vi "dfd_Generate Quantized Gain Report.vi"(8 "error in (no error)":errorcluster, 11 "filter in":T1={"mSRate_Fs"=1.0, "mSRate_Version"="1.0", "mSRate_Comments"="", "mSRate_OrgCoef"={"type"=enum."Undefined", "gain"=1.0, "coef a (k)"=[], "coef b (v)"=[]}, "mSRate_CurCoef"={"type"=enum."Undefined", "gain"=1.0, "coef a (k)"=[], "coef b (v)"=[]}, "mSRate_Quantized?"=FALSE, "mSRate_QCoef"={"type"=enum."Undefined", "gain"=1.0, "coef a (k)"=[], "coef b (v)"=[]}, "mSRate_QSettings"=[], "mSRate_Order"=0, "mSRate_Scaling"={"mSRate_ScaleByPowerOf2?"=FALSE, "mSRate_ScaleType"=enum."No Norm"}} {"mSRate_QSettings"."source" items=["Coef a/k"=0, "Coef b/v"=7, "Input"=1, "Output"=2, "Multiplicand"=3, "Product"=4, "Sum"=5, "Delay"=6, "Gain"=8]}) -> (0 "error out":errorcluster, 2 "gain report":string, 3 "filter out":T1={"mSRate_Fs"=1.0, "mSRate_Version"="1.0", "mSRate_Comments"="", "mSRate_OrgCoef"={"type"=enum."Undefined", "gain"=1.0, "coef a (k)"=[], "coef b (v)"=[]}, "mSRate_CurCoef"={"type"=enum."Undefined", "gain"=1.0, "coef a (k)"=[], "coef b (v)"=[]}, "mSRate_Quantized?"=FALSE, "mSRate_QCoef"={"type"=enum."Undefined", "gain"=1.0, "coef a (k)"=[], "coef b (v)"=[]}, "mSRate_QSettings"=[], "mSRate_Order"=0, "mSRate_Scaling"={"mSRate_ScaleByPowerOf2?"=FALSE, "mSRate_ScaleType"=enum."No Norm"}} {"mSRate_QSettings"."source" items=["Coef a/k"=0, "Coef b/v"=7, "Input"=1, "Output"=2, "Multiplicand"=3, "Product"=4, "Sum"=5, "Delay"=6, "Gain"=8]})   [LabVIEW 2017, in "NI_DigFilter_FXP.lvlib"]
uses:
  <vilib>/addons/Digital Filter Design/NI_DigFilter_FXP.lvlib
  <vilib>/addons/Digital Filter Design/_Objects.llb/DFD Filter Obj.ctl
  <vilib>/addons/Digital Filter Design/_Objects.llb/DFD Filter Coef.ctl
  <vilib>/addons/Digital Filter Design/_Objects.llb/DFD Filter Structure Type Selector.ctl
  <vilib>/addons/Digital Filter Design/_Objects.llb/dfd_Internal Quantization Settings.ctl
  <vilib>/addons/Digital Filter Design/_Objects.llb/dfd_Internal Quantization Srcs.ctl
  <vilib>/addons/Digital Filter Design/_Objects.llb/DFD Coef Norm Type.ctl
  <vilib>/addons/Digital Filter Design/NI_DigFilterLicensed.lvlib
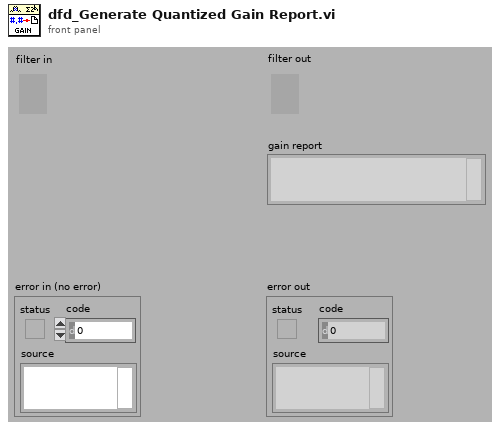
[diagram p1: front panel]
types:
  T1 = typedef "NI_DigFilterLicensed.lvlib/DFD Filter Obj.ctl" = cluster{"mSRate_Fs":dbl, "mSRate_Version":string, "mSRate_Comments":string, "mSRate_OrgCoef":T2, "mSRate_CurCoef":T2, "mSRate_Quantized?":bool, "mSRate_QCoef":T2, "mSRate_QSettings":T4[], "mSRate_Order":i32, "mSRate_Scaling":cluster{"mSRate_ScaleByPowerOf2?":bool, "mSRate_ScaleType":T6}}
  T2 = typedef "NI_DigFilterLicensed.lvlib/DFD Filter Coef.ctl" = cluster{"type":T3, "gain":dbl, "coef a (k)":dbl[], "coef b (v)":dbl[]}
  T3 = typedef "NI_DigFilterLicensed.lvlib/DFD Filter Structure Type Selector.ctl" = enum16{"Undefined", "FIR Direct Form", "FIR Direct Form Transposed", "FIR Symmetric", "FIR Antisymmetric", "IIR Direct Form I", "IIR Direct Form I Transposed", "IIR Direct Form II", "IIR Direct Form II Transposed", "IIR Cascaded Second Order Sections Form I", "IIR Cascaded Second Order Sections Form I Transposed", "IIR Cascaded Second Order Sections Form II", "IIR Cascaded Second Order Sections Form II Transposed", "Lattice Allpass (basic sections)", "Lattice Allpass (one multiplier sections)", "Lattice Allpass (normalized sections)", "Lattice AR (basic sections)", "Lattice AR (one multiplier sections)", "Lattice AR (normalized sections)", "Lattice MA (minimum phase)", "Lattice MA (maximum phase)", "Lattice ARMA (basic sections)", "Lattice ARMA (one multiplier sections)", "Lattice ARMA (normalized sections)"}
  T4 = typedef "NI_DigFilterLicensed.lvlib/dfd_Internal Quantization Settings.ctl" = cluster{"source":T5, "wl":i16, "iwl":i16, "overflow mode":enum16{"Saturation", "Wrap"}, "rounding mode":enum16{"Nearest", "Truncation"}, "signed?":bool}
  T5 = typedef "NI_DigFilterLicensed.lvlib/dfd_Internal Quantization Srcs.ctl" = u16
  T6 = typedef "NI_DigFilterLicensed.lvlib/DFD Coef Norm Type.ctl" = enum16{"No Norm", "Time Domain 1-Norm", "Time Domain 2-Norm", "Time Domain Inf-Norm"}
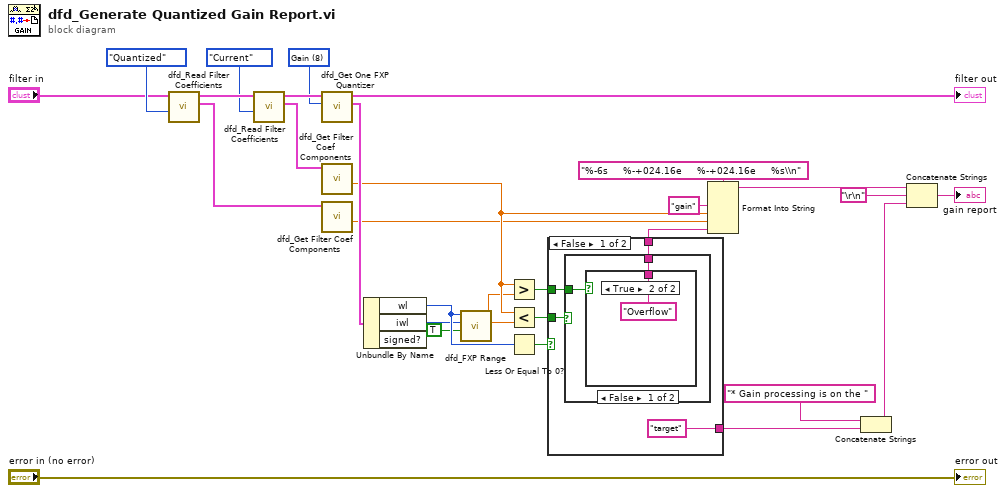
[diagram p0: block diagram]
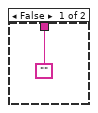
[diagram p2: hidden frame]
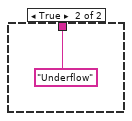
[diagram p3: hidden frame]
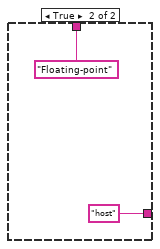
[diagram p4: hidden frame]
diagram:
  w19 = T5 8 items=["Coef a/k"=0, "Coef b/v"=7, "Input"=1, "Output"=2, "Multiplicand"=3, "Product"=4, "Sum"=5, "Delay"=6, "Gain"=8] ("quantization source")
  n1 = call <vilib>:"dfd_Read Filter Coefficients.vi"("coef source"=enum16{"Original", "Current", "Quantized"}."Quantized", "filter in"="filter in") -> ("filter coef"=w24:T2, "filter out"=w30:T1)  [unwired: 1 in, 7 out]
  n2 = call <vilib>:"dfd_Read Filter Coefficients.vi"("coef source"=enum16{"Original", "Current", "Quantized"}."Current", "filter in"=w30) -> ("filter coef"=w26:T2, "filter out"=w29:T1)  [unwired: 1 in, 7 out]
  n3 = call <vilib>:"dfd_Get One FXP Quantizer.vi"("quantization source"=w19, "filter in"=w29) -> ("quantization settings"=w23:T4, "filter out"=→"filter out":T1)  [unwired: 1 in, 7 out]
  n4 = call <vilib>:"dfd_Get Filter Coef Components.vi"("filter coef"=w26) -> ("gain"=w22:dbl)  [unwired: 1 in, 9 out]
  n5 = call <vilib>:"dfd_Get Filter Coef Components.vi"("filter coef"=w24) -> ("gain"=w21:dbl)  [unwired: 1 in, 9 out]
  n6 = Unbundle By Name(w23) -> ("wl"=w4:i16, "iwl"=w3:i16)  [unwired: 1 out]
  n7 = call <vilib>:"dfd_FXP Range.vi"("signed?"=TRUE, "iwl"=w3, "wl"=w4) -> ("low"=w18:ext, "high"=w17:ext)  [unwired: 7 out]
  n8 = Greater?(x=w22, y=w17) -> (0:w11:bool)
  n9 = Less?(x=w22, y=w18) -> (x < y?=w14:bool)
  n10 = Less Or Equal To 0?(x=w4) -> (x <= 0?=w12:bool)
  n11 = case shown="False" w12 {
    tunnel: w14 -> [w34 _]
    tunnel: [w33 "Floating-point"] -> w13
    tunnel: w11 -> [w32 _]
    tunnel: ["target" "host"] -> w9
    frame False {
      n12 = case shown="False" w34 {
        tunnel: [w36 "Underflow"] -> w33
        tunnel: w32 -> [w35 _]
        frame False {
          n13 = case shown="True" w35 {
            tunnel: ["" "Overflow"] -> w36
            frame False {
            }
            frame True {
            }
          }
        }
        frame True {
        }
      }
    }
    frame True {
    }
  }
  n14 = Format Into String(format string="%-6s     %-+024.16e     %-+024.16e     %s\\n", "gain" ("input 1"), w22, w21, w13) -> (resulting string=w6:string)  [unwired: 2 in, 1 out]
  n15 = Concatenate Strings("* Gain processing is on the " ("string"), w9) -> (w7:string)
  n16 = Concatenate Strings(w6, "\r\n", w7) -> (→"gain report":string)
  "error out" <- "error in (no error)"
